vi "ChapR TH Translate.vi"(11 "Tophat Value":u8) -> (1 "Y":i8, 2 "X":i8)   [LabVIEW 2013]
doc: "Changes the tophat values (integers 0 to 7 inclusive) to the x and y axes (integers -127 to 127).\n\n*the tophat is the little plus sign thingy on the controller"
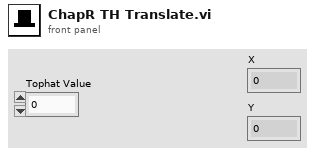
[diagram p1: front panel]
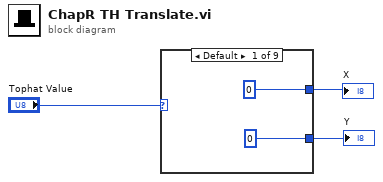
[diagram p0: block diagram]
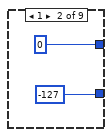
[diagram p2: hidden frame]
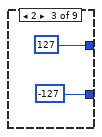
[diagram p3: hidden frame]
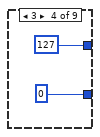
[diagram p4: hidden frame]
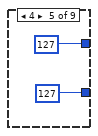
[diagram p5: hidden frame]
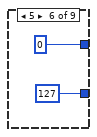
[diagram p6: hidden frame]
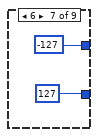
[diagram p7: hidden frame]
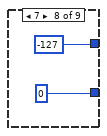
[diagram p8: hidden frame]
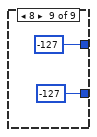
[diagram p9: hidden frame]
diagram:
  n1 = case shown="Default" "Tophat Value" {
    tunnel: [i8 0 i8 0 i8 127 i8 127 i8 127 i8 0 i8 -127 i8 -127 i8 -127] -> w2
    tunnel: [i8 0 i8 -127 i8 -127 i8 0 i8 127 i8 127 i8 127 i8 0 i8 -127] -> w1
    frame Default {
    }
    frame 1 {
    }
    frame 2 {
    }
    frame 3 {
    }
    frame 4 {
    }
    frame 5 {
    }
    frame 6 {
    }
    frame 7 {
    }
    frame 8 {
    }
  }
  "Y" <- w1
  "X" <- w2
